vi "H5Fopen.vi"(5 "access_id":T1, 6 "error in (no error)":errorcluster, 7 "flags":u32(ring)=1 items=["H5F_ACC_RDONLY", "H5F_ACC_RDWR"], 9 "path":path) -> (0 "error out":errorcluster, 3 "HDF5 Ref out":T1)   [LabVIEW 2017]
doc: "Opens an existing HDF5 file."
uses:
  <vilib>/UPVI/lvhdf5/library.llb/HDF5 Ref.ctl
  <vilib>/UPVI/lvhdf5/hdf5.dll
panel:
  # "LVHDF5 Toolkit\nCopyright (c) 2005-2013 by Jason D. Sommerville\nCopyright (c) 2014 by UPVI, LLC.\n\nThis use and distribution of this file is governed by the terms found in \nLICENSE.txt distributed with this toolkit and installed at\n <user.lib>\\_lvhdf5\\LICENSE.txt"
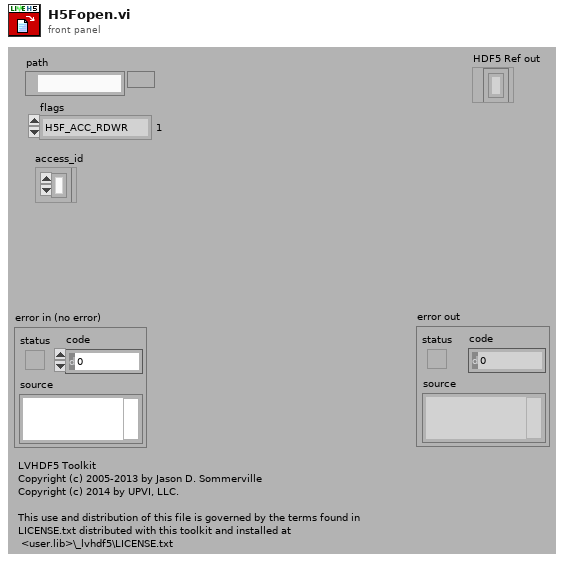
[diagram p1: front panel]
types:
  T1 = typedef "HDF5 Ref.ctl" = refnum<k1>
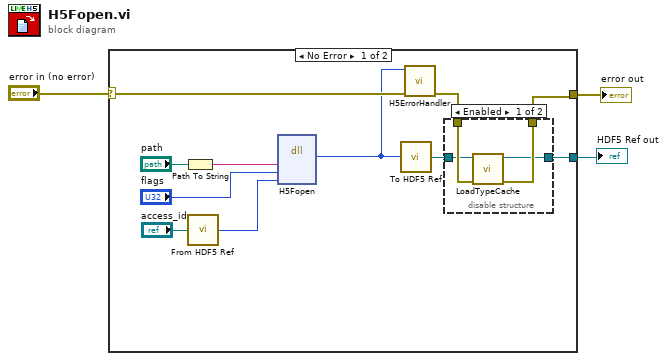
[diagram p0: block diagram]
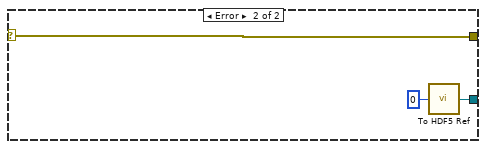
[diagram p3: hidden frame]
diagram:
  n1 = case shown="No Error" "error in (no error)" {
    selector: "error in (no error)" -> [w14 w23]
    tunnel: [w6 w23] -> w2
    tunnel: [w4 w22] -> w1
    frame No Error {
      n2 = Path To String(path="path") -> (string=w13:string)
      n3 = call <vilib>:"From HDF5 Ref.vi"("HDF5 Ref"="access_id") -> ("I32"=w9:i32)
      n4 = dll-call lib="C:/Program Files/National Instruments/LabVIEW 2017/vi.lib/UPVI/lvhdf5/hdf5.dll" fn="H5Fopen"("path"=w13, "flags"="flags", "access_id"=w9) -> ("return type"=w8:i32)  [unwired: 6 in, 2 out]
      n5 = call <vilib>:"To HDF5 Ref.vi"("I32"=w8) -> ("HDF5 Ref"=w5:T1)
      n6 = call <vilib>:"H5ErrorHandler.vi"("error in (no error)"=w14, "herr_t"=w8) -> ("error out"=w7:errorcluster)  [unwired: 3 in, 4 out]
      n7 = disable-structure shown="Enabled" {
        disable-tunnel: w7 -> [w18 w19]
        disable-tunnel: [w17 w19] -> w6
        disable-tunnel: w5 -> [w16 w20]
        disable-tunnel: [w15 w20] -> w4
        frame Enabled {
          n8 = call <vilib>:"LoadTypeCache.vi"("error in (no error)"=w18, "Any HDF5 Refnum"=w16) -> ("error out"=w17:errorcluster, "Any HDF5 Refnum out"=w15:T1)  [unwired: 7 in, 1 out]
        }
        frame Disabled {
        }
      }
    }
    frame Error {
      n9 = call <vilib>:"To HDF5 Ref.vi"("I32"=0) -> ("HDF5 Ref"=w22:T1)
    }
  }
  "error out" <- w2
  "HDF5 Ref out" <- w1
